vi "libssh2_knownhost_init - invalid session - returns invalid known hosts collection.vi"() -> ()   [LabVIEW 2017, in "unit_tests.lvlib"]
uses:
  unit_tests.lvlib
  libssh2/Session Refnum.ctl
  libssh2/libssh2_init_default.vi
  libssh2/libssh2.lvlib
  <vilib>/PNR/Transparent Assertions/Transparent Assertions/Transparent Assertions.lvlib
panel:
  out "error out":errorcluster
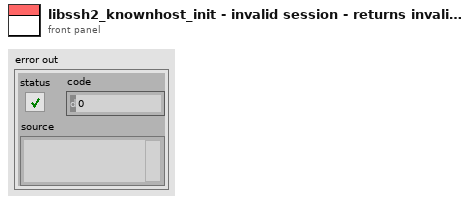
[diagram p1: front panel]
types:
  T1 = typedef "libssh2.lvlib/Session Refnum.ctl" = refnum<k1>
  T2 = typedef "libssh2.lvlib/Host Key Database Refnum.ctl" = refnum<k1>
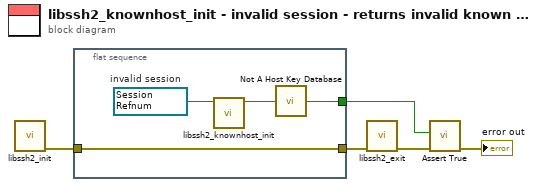
[diagram p0: block diagram]
diagram:
  n1 = call-poly "libssh2_init.vi"() -> ("error out"=w1:errorcluster)  [unwired: 11 in]
  n2 = flat-sequence {
    tunnel: [w9] -> w3
    tunnel: [w8] -> w2
    tunnel: w1 -> [w8]
    frame #0 {
      w7 = T1 refnum items=["Session"]  # invalid session
      n3 = call "libssh2_knownhost_init.vi"("session"=w7) -> ("host key database"=w6:T2)  [unwired: 9 in, 1 out]
      n4 = call "Not A Host Key Database.vi"("host key database"=w6) -> ("Not a Host Key Database?"=w9:bool)
    }
  }
  n5 = call "libssh2_exit.vi"("error in (no error)"=w2) -> ("error out"=w4:errorcluster)  [unwired: 10 in]
  n6 = call <vilib>:"Assert True.vi"("error in (no error)"=w4, "Condition"=w3) -> ("error out"=→"error out":errorcluster)  [unwired: 9 in]
